vi "Open.vi"(8 "error in (no error)":errorcluster) -> (0 "error out":errorcluster, 3 "Refnum":refnum<k7>)   [LabVIEW 2020, in "lvpptx.lvlib"]
uses:
  lvpptx.lvlib
panel:
  # "Connect to PPT and return refnum"
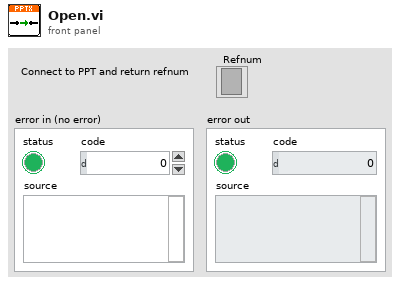
[diagram p1: front panel]
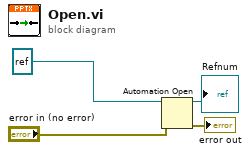
[diagram p0: block diagram]
diagram:
  n1 = Automation Open(error in (no error)="error in (no error)", Automation Refnum=refnum<k7> refnum ("PowerPoint._Application")) -> (Automation Refnum=→"Refnum":refnum<k7>, error out=→"error out":errorcluster)  [unwired: 2 in]
